vi "Source Measure and Visualize.vi"() -> ()   [LabVIEW 2021]
uses:
  <instrlib>/niDCPower/nidcpower.llb/niDCPower Source Mode.ctl
  <instrlib>/niDCPower/nidcpower.llb/niDCPower Output Function.ctl
  <instrlib>/Agilent 3446X Series/Public/Data/Read (Single Point).vi
  <instrlib>/Agilent 3446X Series/Agilent 3446X Series.lvlib
  <instrlib>/Tektronix MSO5X Series/Tektronix MSO5X Series.lvlib
panel:
  in  "Maximum Record Length":dbl=250000000.0 format="%#_6e"
  in  "Sample Rate":dbl=3125000000.0
  in  "Control Type":i32(ring) items=["Horizontal Scale", "Record Length"]
  out "Division Number":i32
  out "Timebase Duration (s)":dbl
  out "Interpolation Ratio":dbl
  in  "Keithley Scope":refnum<visa-resource-name>
  in  "Absolute Resolution (1E-6)":dbl=1e-06
  in  "Agilent DMM":refnum<visa-resource-name>
  in  "Manual Range (1)":dbl=1.0
  out "Measurement using DMM":dbl
  in  "error in":errorcluster
  out "error out":errorcluster
  out "Voltage Measurement":dbl
  out "Current Measurement":dbl
  in  "Current Limit":dbl=0.01 format="%.3p"
  in  "Voltage Level":dbl=2.0 format="%.5p"
  in  "Vin SMU Channel":string="0"
  in  "Vin SMU":refnum<k15>="Dev1"
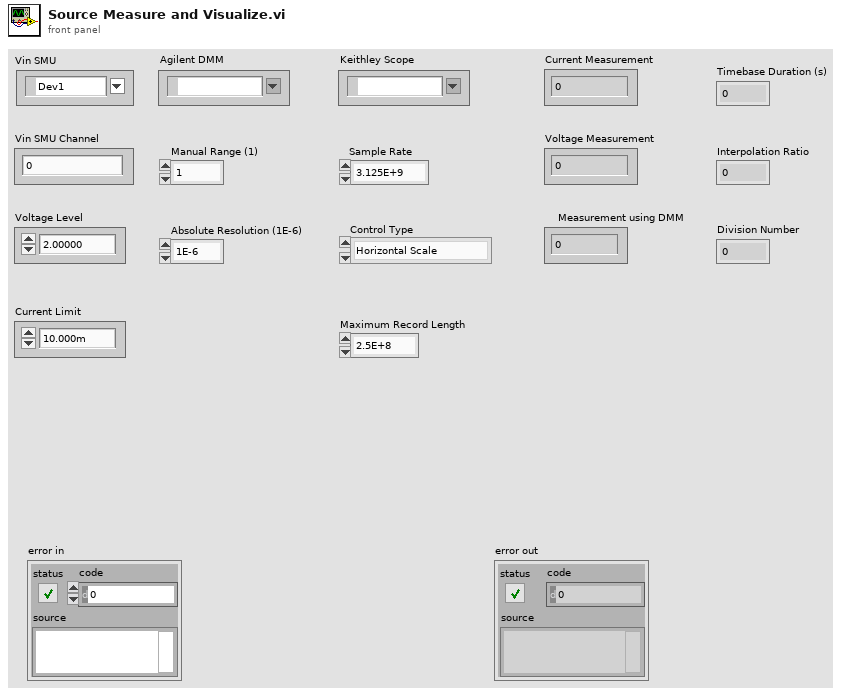
[diagram p1: front panel]
types:
  T1 = typedef "niDCPower Output Function.ctl" = i32
  T2 = typedef "niDCPower Source Mode.ctl" = i32
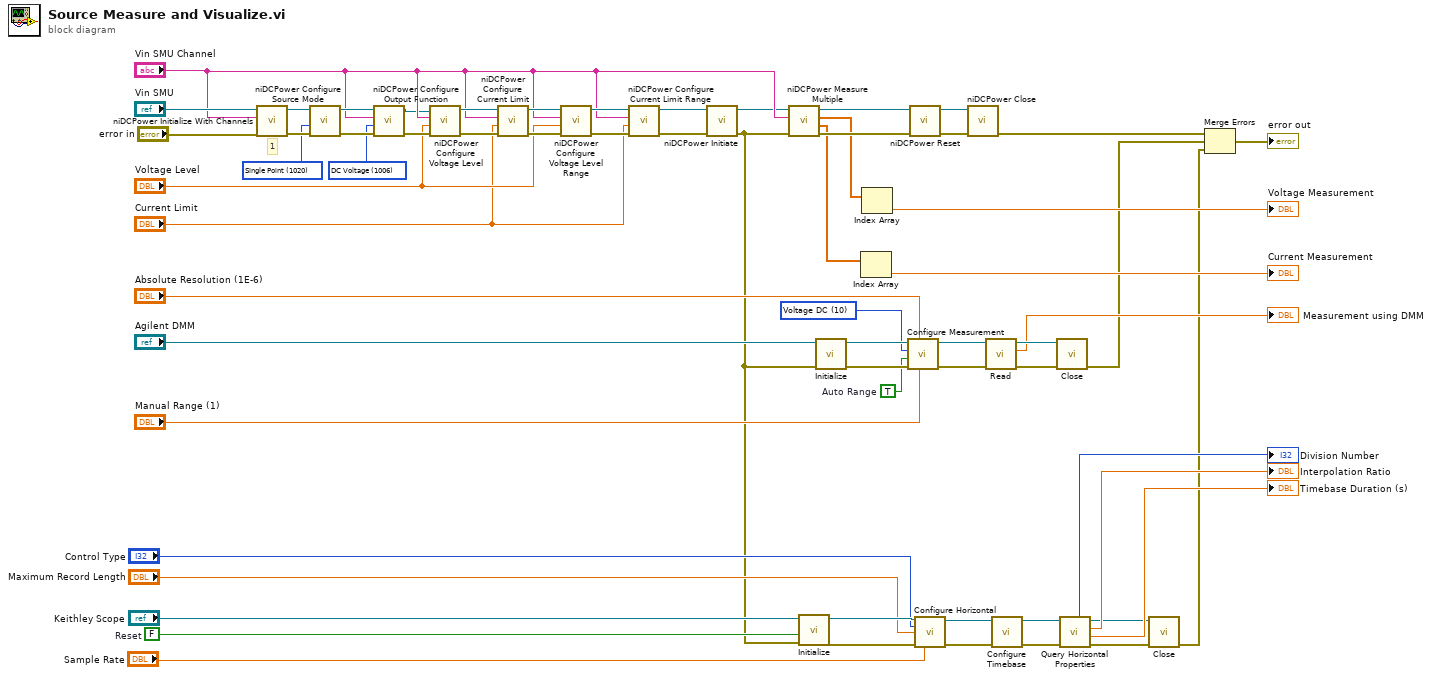
[diagram p0: block diagram]
diagram:
  w19 = FALSE  # Reset
  w21 = TRUE  # Auto Range
  w24 = 10 items=["Continuity", "Current AC", "Current DC", "Diode", "Frequency", "Resistance 4-wire", "Period", "Resistance 2-wire", "Temperature", "Voltage AC", "Voltage DC", "Voltage DC Ratio", "Capacitance"] ("Measurement Function (10: Voltage DC)")
  w41 = T1 1006 items=["DC Voltage"=1006, "DC Current"=1007, "Pulse Voltage"=1049, "Pulse Current"=1050] ("output function")
  w54 = T2 1020 items=["Single Point"=1020, "Sequence"=1021] ("source mode")
  # "1"
  n1 = call <instrlib>:"niDCPower Initialize With Channels.vi"("error in (no error)"="error in", "channels"="Vin SMU Channel", "resource name"="Vin SMU") -> ("error out"=w58:errorcluster, "instrument handle out"=w57:refnum<k15>)  [unwired: 2 in, 5 out]
  n2 = call <instrlib>:"niDCPower Configure Source Mode.vi"("error in (no error)"=w58, "source mode"=w54, "instrument handle"=w57) -> ("error out"=w56:errorcluster, "instrument handle out"=w55:refnum<k15>)  [unwired: 7 out]
  n3 = call <instrlib>:"niDCPower Configure Output Function.vi"("error in (no error)"=w56, "output function"=w41, "channel name"="Vin SMU Channel", "instrument handle"=w55) -> ("error out"=w42:errorcluster, "instrument handle out"=w43:refnum<k15>)  [unwired: 6 out]
  n4 = call <instrlib>:"niDCPower Configure Voltage Level.vi"("error in (no error)"=w42, "voltage level"="Voltage Level", "channel name"="Vin SMU Channel", "instrument handle"=w43) -> ("error out"=w61:errorcluster, "instrument handle out"=w62:refnum<k15>)  [unwired: 6 out]
  n5 = call <instrlib>:"niDCPower Configure Current Limit.vi"("error in (no error)"=w61, "current limit"="Current Limit", "channel name"="Vin SMU Channel", "instrument handle"=w62) -> ("error out"=w53:errorcluster, "instrument handle out"=w52:refnum<k15>)  [unwired: 1 in, 5 out]
  n6 = call <instrlib>:"niDCPower Configure Voltage Level Range.vi"("error in (no error)"=w53, "voltage level range"="Voltage Level", "channel name"="Vin SMU Channel", "instrument handle"=w52) -> ("error out"=w51:errorcluster, "instrument handle out"=w50:refnum<k15>)  [unwired: 6 out]
  n7 = call <instrlib>:"niDCPower Configure Current Limit Range.vi"("error in (no error)"=w51, "current limit range"="Current Limit", "channel name"="Vin SMU Channel", "instrument handle"=w50) -> ("error out"=w46:errorcluster, "instrument handle out"=w47:refnum<k15>)  [unwired: 6 out]
  n8 = call <instrlib>:"niDCPower Initiate.vi"("error in (no error)"=w46, "instrument handle"=w47) -> ("error out"=w3:errorcluster, "instrument handle out"=w44:refnum<k15>)  [unwired: 2 in, 6 out]
  n9 = call <instrlib>:"niDCPower Measure Multiple.vi"("error in (no error)"=w3, "channel name"="Vin SMU Channel", "instrument handle"=w44) -> ("error out"=w48:errorcluster, "current measurements"=w38:dbl[], "voltage measurements"=w36:dbl[], "instrument handle out"=w49:refnum<k15>)  [unwired: 5 out]
  n10 = call <instrlib>:"Initialize.vi"("error in (no error)"=w3, "Reset (True)"=w19, "VISA resource name"="Keithley Scope") -> ("error out"=w17:errorcluster, "VISA resource name out"=w18:refnum<visa-resource-name>)  [unwired: 7 in]
  n11 = call <instrlib>:"Initialize.vi"("error in (no error)"=w3, "VISA resource name"="Agilent DMM") -> ("error out"=w33:errorcluster, "VISA resource name out"=w34:refnum<visa-resource-name>)  [unwired: 3 in, 5 out]
  n12 = Index Array(array=w38) -> (element=→"Current Measurement":dbl)  [unwired: 1 in]
  n13 = Index Array(array=w36) -> (element=→"Voltage Measurement":dbl)  [unwired: 1 in]
  n14 = call <instrlib>:"Configure Measurement.vi"("Manual Range (1)"="Manual Range (1)", "Absolute Resolution (1E-6)"="Absolute Resolution (1E-6)", "error in (no error)"=w33, "Auto Range (T: Enable)"=w21, "Measurement Function (10: Voltage DC)"=w24, "VISA resource name"=w34) -> ("error out"=w29:errorcluster, "VISA resource name out"=w30:refnum<visa-resource-name>)  [unwired: 4 out]
  n15 = call <instrlib>:"niDCPower Reset.vi"("error in (no error)"=w48, "instrument handle"=w49) -> ("error out"=w59:errorcluster, "instrument handle out"=w60:refnum<k15>)  [unwired: 2 in, 6 out]
  n16 = call <instrlib>:"Configure Horizontal.vi"("VISA resource name"=w18, "Control Type (0: Horizontal Scale)"="Control Type", "Maximum Record Length (2.5E+8)"="Maximum Record Length", "error in (no error)"=w17, "Sample Rate (3.125E+9)"="Sample Rate") -> ("VISA resource name out"=w8:refnum<visa-resource-name>, "error out"=w7:errorcluster)  [unwired: 9 in]
  n17 = call <instrlib>:"niDCPower Close.vi"("error in (no error)"=w59, "instrument handle"=w60) -> ("error out"=w39:errorcluster)  [unwired: 9 out]
  n18 = call-poly <instrlib>:"Read.vi"("error in (no error)"=w29, "VISA resource name"=w30) -> ("error out"=w32:errorcluster, "Measurement"=→"Measurement using DMM":dbl, "VISA resource name out"=w31:refnum<visa-resource-name>)  [unwired: 7 out]
  n19 = call <instrlib>:"Configure Timebase.vi"("error in (no error)"=w7, "VISA resource name"=w8) -> ("error out"=w6:errorcluster, "VISA resource name out"=w5:refnum<visa-resource-name>)  [unwired: 8 in]
  n20 = call <instrlib>:"Close.vi"("error in (no error)"=w32, "VISA resource name"=w31) -> ("error out"=w22:errorcluster)  [unwired: 9 out]
  n21 = call <instrlib>:"Query Horizontal Properties.vi"("error in (no error)"=w6, "VISA resource name"=w5) -> ("error out"=w9:errorcluster, "Timebase Duration (s)"=→"Timebase Duration (s)":dbl, "Interpolation Ratio"=→"Interpolation Ratio":dbl, "VISA resource name out"=w10:refnum<visa-resource-name>, "Division Number"=→"Division Number":i32)  [unwired: 5 in]
  n22 = call <instrlib>:"Close.vi"("error in (no error)"=w9, "VISA resource name"=w10) -> ("error out"=w4:errorcluster)  [unwired: 9 in]
  n23 = Merge Errors(w39, w22, w4) -> (→"error out":errorcluster)
